vi "2D Lobatto Quadrature Core.vi"(6 "VI ref":cluster{"f(X)":refnum<vi>, "data":variant}, 7 "formula":string, 9 "tolerance":dbl=1e-10, 10 "Formula/VI ref":bool, 11 "limits":T1={"x limit"={"x lower"=0.0, "x upper"=1.0}, "y limit"={"y lower"=0.0, "y upper"=1.0}}) -> (0 "error out":errorcluster, 3 "result":dbl)   [LabVIEW 2018, in "NI_AALPro.lvlib"]
uses:
  NI_AALPro.lvlib
  A x Vector.vi
  Real Dot Product.vi
  NI_AALBase.lvlib
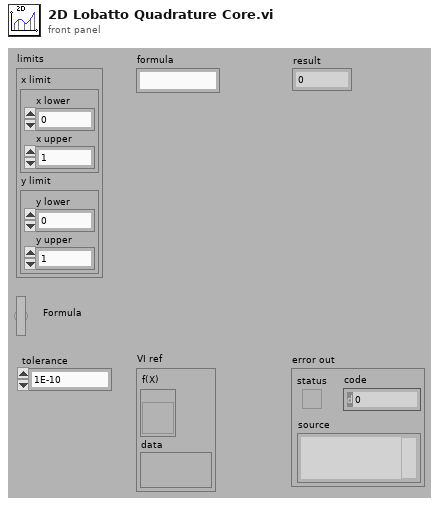
[diagram p1: front panel]
types:
  T1 = cluster{"x limit":cluster{"x lower":dbl, "x upper":dbl}, "y limit":cluster{"y lower":dbl, "y upper":dbl}}
  T2 = cluster{string[], "Variable Output":string, "formula":string}
  T3 = cluster{"x limit":cluster{"x lower":dbl, "x upper":dbl}, "y limit":cluster{"y lower":dbl, "y upper":dbl}}[]
  T4 = cluster{"bin x":cluster{"lower limit":dbl, "upper limit":dbl}, "bin y":cluster{"lower limit":dbl, "upper limit":dbl}}[]
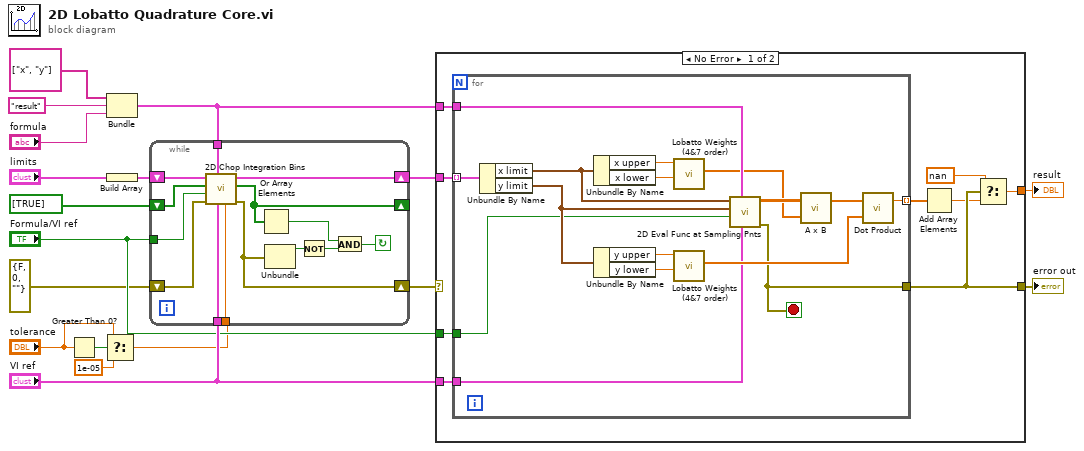
[diagram p0: block diagram]
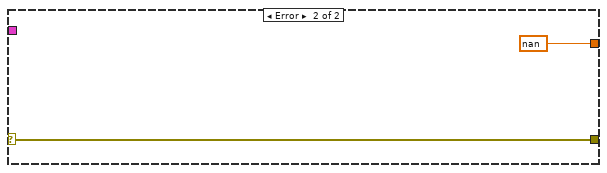
[diagram p2: hidden frame]
diagram:
  n1 = Greater Than 0?(x="tolerance") -> (x > 0?=w5:bool)
  n2 = Select(t="tolerance", s=w5, f=1e-05) -> (s? t:f=w2:dbl)
  n3 = Bundle(string[] ["x", "y"], "Variable Output"="result", "formula"="formula") -> (w9:T2)  [unwired: 1 out]
  n4 = Build Array("limits") -> (w18:T3)
  n5 = while {
    shift-right: [w31] -> w15
    shift-left: w18 -> [w32]
    shift-right: [w29] -> _
    shift-left: bool[] [TRUE] ("appended array") -> [w30]
    tunnel: w9 -> [w25]
    tunnel: "Formula/VI ref" -> [w28]
    tunnel: "VI ref" -> [w27]
    tunnel: w2 -> [w26]
    shift-right: [w21] -> w1
    shift-left: errorcluster {"status"=FALSE, "code"=0, "source"=""} ("error out") -> [w24]
    stop <- w19 continue-if-true
    n6 = call "2D Chop Integration Bins.vi"("tolerance"=w26, "VI ref"=w27, "Formula"=w25, "error in (no error)"=w24, "Formula/VI ref"=w28, "Chop In"=w30, "Bins In"=w32) -> ("error out"=w21:errorcluster, "Chop Out"=w29:bool[], "Bins Out"=w31:T4)  [unwired: 2 out]
    n7 = Or Array Elements(Boolean array=w29) -> (logical OR=w20:bool)
    n8 = Unbundle(w21) -> ("status"=w23:bool)  [unwired: 2 out]
    n9 = Not(x=w23) -> (.not. x?=w22:bool)
    n10 = And(x=w20, y=w22) -> (x .and. y?=w19:bool)
  }
  n11 = case shown="No Error" w1 {
    selector: w1 -> [_ w59]
    tunnel: [w33 nan ("X * Y")] -> w17
    tunnel: w15 -> [w41 _]
    tunnel: [w36 w59] -> w14
    tunnel: w9 -> [w39 _]
    tunnel: "VI ref" -> [w38 _]
    tunnel: "Formula/VI ref" -> [w37 _]
    frame No Error {
      n12 = for {
        tunnel: w41 -> [w57] mode=indexing
        tunnel: [w51] -> w40 mode=indexing
        tunnel: w37 -> [w48]
        tunnel: w38 -> [w47]
        tunnel: w39 -> [w46]
        tunnel: [w45] -> w36
        stop <- w45 stop-if-true
        n13 = Unbundle By Name(w57) -> ("x limit"=w56:cluster{"x lower":dbl, "x upper":dbl}, "y limit"=w55:cluster{"y lower":dbl, "y upper":dbl})
        n14 = Unbundle By Name(w56) -> ("x upper"=w50:dbl, "x lower"=w49:dbl)
        n15 = Unbundle By Name(w55) -> ("y upper"=w54:dbl, "y lower"=w53:dbl)
        n16 = call "Lobatto Weights (4&7 order).vi"("lower limit"=w49, "upper limit"=w50) -> ("Weights (7-Order)"=w43:dbl[])  [unwired: 9 out]
        n17 = call "Lobatto Weights (4&7 order).vi"("lower limit"=w53, "upper limit"=w54) -> ("Weights (7-Order)"=w52:dbl[])  [unwired: 9 out]
        n18 = call "2D Eval Func at Sampling Pnts.vi"("VI ref"=w47, "Formula"=w46, "Formula/VI ref"=w48, "y limit"=w55, "x limit"=w56) -> ("error out"=w45:errorcluster, "Function Evaluations (7 pts)"=w44:dbl[][])  [unwired: 1 in, 4 out]
        n19 = call-poly "A x B.vi"("Vector"=w43, "A"=w44) -> ("A x Vector"=w42:dbl[])  [unwired: 1 out]
        n20 = call-poly "Dot Product.vi"("Y Vector"=w52, "X Vector"=w42) -> ("X * Y"=w51:dbl)  [unwired: 1 out]
      }
      n21 = Add Array Elements(numeric array=w40) -> (sum=w35:dbl)
      n22 = Select(t=nan, s=w36, f=w35) -> (s? t:f=w33:dbl)
    }
    frame Error {
    }
  }
  "result" <- w17
  "error out" <- w14
